vi "Tree_Pathnames_to_create.vi"(2 "Precision":i32[](array[numeric]), 3 "Tree Root":path, 4 "Channel Values In":string[][](array[string]), 5 "Ch names In":string[](array[string]), 6 "Tree channel Tolerances":dbl[](array[numeric]) format="%.2f", 7 "Tree channel Indicies":i32[](array[numeric])) -> (1 "Filenames to append to":path[](array[path]))   [LabVIEW 2010]
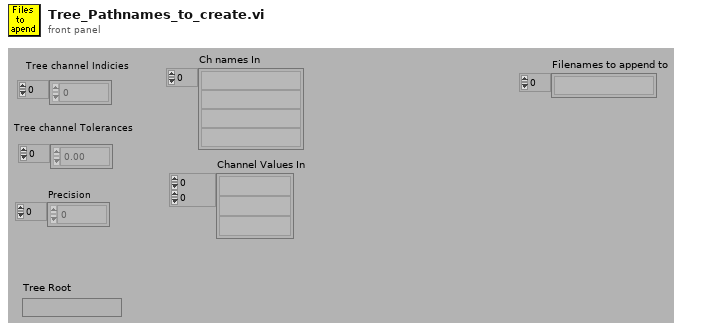
[diagram p1: front panel]
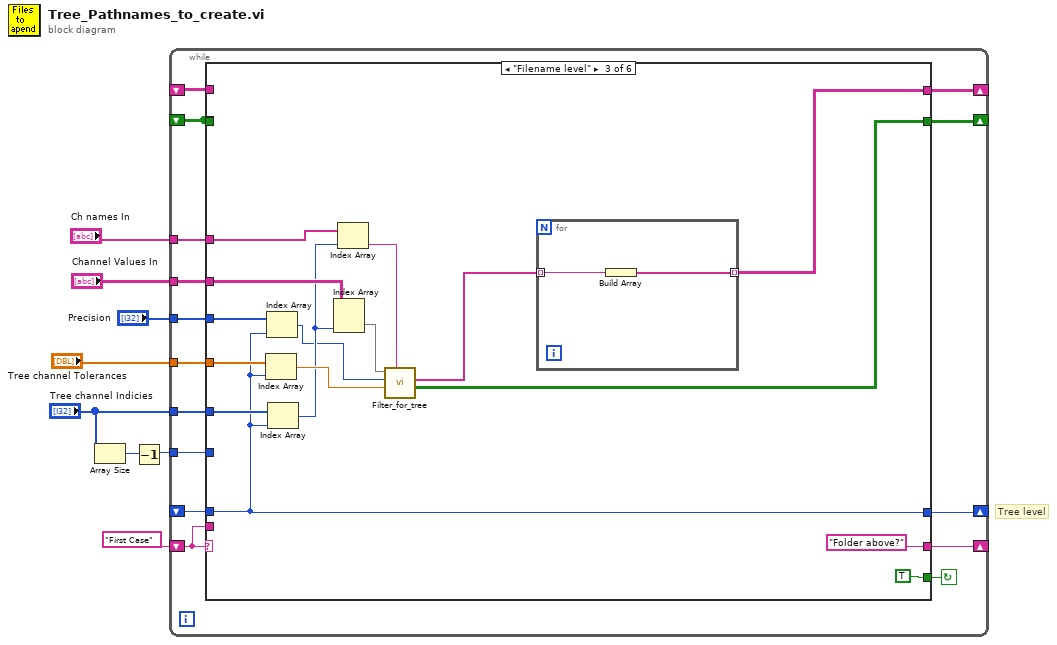
[diagram p0: block diagram]
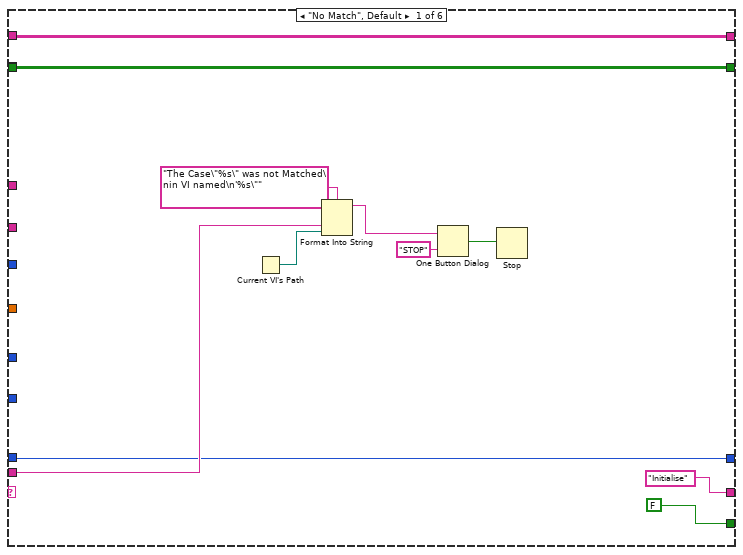
[diagram p2: hidden frame]
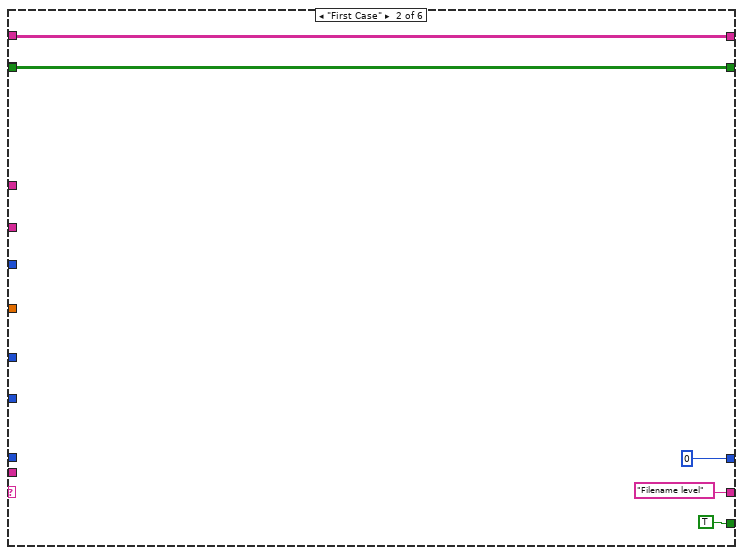
[diagram p3: hidden frame]
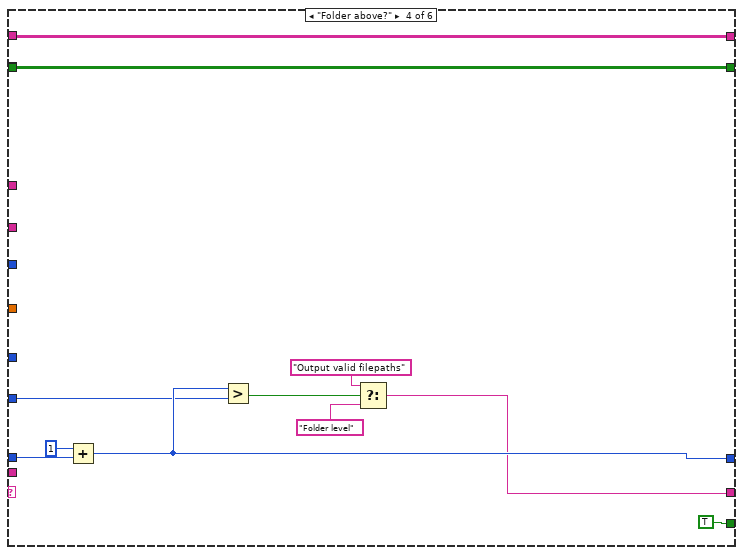
[diagram p4: hidden frame]
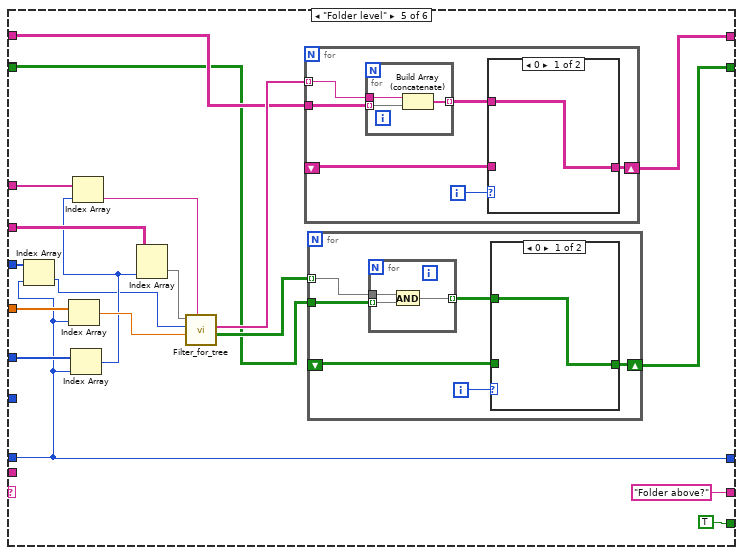
[diagram p5: hidden frame]
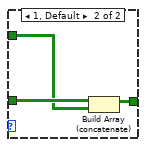
[diagram p6: hidden frame]
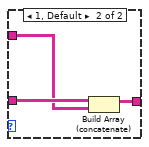
[diagram p7: hidden frame]
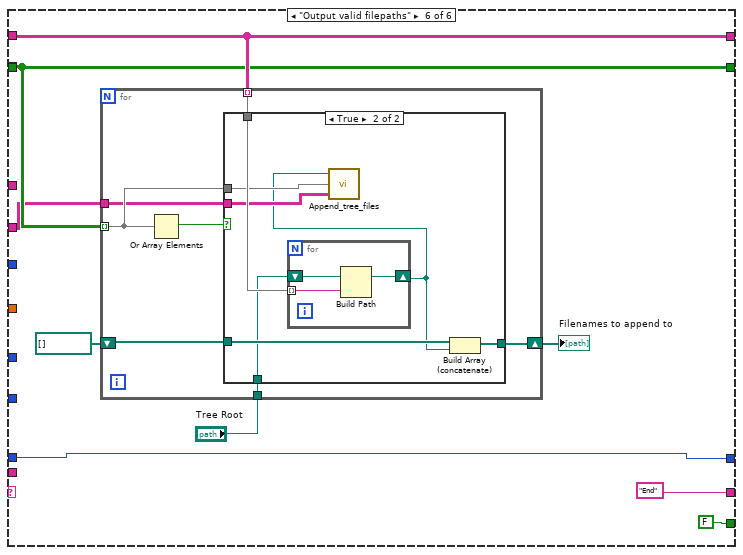
[diagram p8: hidden frame]
diagram:
  # "Tree level"
  n1 = Array Size(array="Tree channel Indicies") -> (size(s)=w4:i32)
  n2 = Decrement(x=w4) -> (x-1=w3:i32)
  n3 = while {
    tunnel: "Precision" -> [w9]
    tunnel: "Ch names In" -> [w10]
    tunnel: w3 -> [w11]
    tunnel: "Channel Values In" -> [w14]
    tunnel: "Tree channel Tolerances" -> [w15]
    shift-left: _ -> [w12]
    shift-right: [w16] -> _
    shift-left: _ -> [w13]
    shift-right: [w17] -> _
    tunnel: "Tree channel Indicies" -> [w18]
    shift-left: _ -> [w19]
    shift-right: [w20] -> _
    shift-left: "First Case" -> [w21]
    shift-right: [w22] -> _
    stop <- w23 continue-if-true
    n4 = case shown="\"Filename level\"" w21 {
      tunnel: [FALSE TRUE TRUE TRUE TRUE FALSE] -> w23
      tunnel: ["Initialise" "Filename level" "Folder above?" w58 "Folder above?" "End"] -> w22
      tunnel: w21 -> [w29 _ _ _ _ _]
      tunnel: [w24 0 w42 w63 w70 w116] -> w20
      tunnel: w19 -> [w24 _ w42 w65 w70 w116]
      tunnel: w18 -> [_ _ w53 _ w86 _]
      tunnel: [w26 w36 w51 w67 w79 w119] -> w17
      tunnel: [w25 w35 w50 w66 w76 w115] -> w16
      tunnel: w15 -> [_ _ w49 _ w84 _]
      tunnel: w14 -> [_ _ w47 _ w82 w114]
      tunnel: w13 -> [w26 w36 _ w67 w80 w119]
      tunnel: w12 -> [_ w35 _ w66 w77 w115]
      tunnel: w12 -> [w25 _ _ _ _ _]
      tunnel: w11 -> [_ _ _ w62 _ _]
      tunnel: w10 -> [_ _ w44 _ w75 _]
      tunnel: w9 -> [_ _ w41 _ w71 _]
      frame "No Match", Default {
        n5 = Current VI's Path() -> (path=w28:path)
        n6 = Format Into String(format string="The Case\"%s\" was not Matched\nin VI named\n'%s\"" ("Format String"), w29, w28) -> (resulting string=w32:string)  [unwired: 2 in, 1 out]
        n7 = One Button Dialog(message=w32, button name ("OK")="STOP") -> (true=w30:bool)
        n8 = Stop(stop? (T)=w30) -> ()
      }
      frame "First Case" {
      }
      frame "Filename level" {
        n9 = Index Array(array=w49, index=w42) -> (element=w48:dbl)
        n10 = Index Array(array=w41, index=w42) -> (element=w40:i32)
        n11 = Index Array(array=w53, index=w42) -> (element=w45:i32)
        n12 = Index Array(array=w47, index (col)=w45) -> (element=w46:string[])  [unwired: 1 in]
        n13 = Index Array(array=w44, index=w45) -> (element=w43:string)
        n14 = call "Filter_for_tree.vi"("Ch Name"=w43, "Tolerance"=w48, "Precision"=w40, "Ch Values In"=w46) -> ("Accept array"=w50:bool[][], "Bin Names"=w52:string[])  [unwired: 4 in]
        n15 = for {
          tunnel: w52 -> [w57] mode=indexing
          tunnel: [w56] -> w51 mode=indexing
          n16 = Build Array(w57) -> (w56:string[])
        }
      }
      frame "Folder above?" {
        n17 = Add(x=1, y=w65) -> (x+y=w63:i32)
        n18 = Greater?(x=w63, y=w62) -> (0:w61:bool)
        n19 = Select(t="Output valid filepaths", s=w61, f="Folder level") -> (s? t:f=w58:string)
      }
      frame "Folder level" {
        n20 = Index Array(array=w71, index=w70) -> (element=w69:i32)
        n21 = Index Array(array=w84, index=w70) -> (element=w83:dbl)
        n22 = Index Array(array=w86, index=w70) -> (element=w73:i32)
        n23 = Index Array(array=w75, index=w73) -> (element=w72:string)
        n24 = Index Array(array=w82, index (col)=w73) -> (element=w81:string[])  [unwired: 1 in]
        n25 = call "Filter_for_tree.vi"("Ch Name"=w72, "Tolerance"=w83, "Precision"=w69, "Ch Values In"=w81) -> ("Accept array"=w78:bool[][], "Bin Names"=w85:string[])  [unwired: 4 in]
        n26 = for {
          tunnel: w85 -> [w106] mode=indexing
          tunnel: w80 -> [w105]
          shift-right: [w103] -> w79
          shift-left: _ -> [w101]
          i -> [w104]
          n27 = for {
            tunnel: w106 -> [w113]
            tunnel: w105 -> [w112] mode=indexing
            tunnel: [w111] -> w102 mode=indexing
            n28 = Build Array (concatenate)(w113, w112) -> (w111:string[])
          }
          n29 = case shown="0" w104 {
            tunnel: [w107 w108] -> w103
            tunnel: w102 -> [w107 w109]
            tunnel: w101 -> [_ w110]
            frame 0 {
            }
            frame 1, Default {
              n30 = Build Array (concatenate)(w110, w109) -> (w108:string[][])
            }
          }
        }
        n31 = for {
          tunnel: w78 -> [w93] mode=indexing
          tunnel: w77 -> [w92]
          shift-right: [w90] -> w76
          shift-left: _ -> [w88]
          i -> [w91]
          n32 = for {
            tunnel: w93 -> [w100]
            tunnel: w92 -> [w99] mode=indexing
            tunnel: [w98] -> w89 mode=indexing
            n33 = And(x=w100, y=w99) -> (x .and. y?=w98:bool[])
          }
          n34 = case shown="0" w91 {
            tunnel: [w94 w95] -> w90
            tunnel: w89 -> [w94 w96]
            tunnel: w88 -> [_ w97]
            frame 0 {
            }
            frame 1, Default {
              n35 = Build Array (concatenate)(w97, w96) -> (w95:bool[][])
            }
          }
        }
      }
      frame "Output valid filepaths" {
        n36 = for {
          tunnel: w115 -> [w124] mode=indexing
          tunnel: "Tree Root" -> [w128]
          tunnel: w119 -> [w127] mode=indexing
          shift-right: [w125] -> w117
          shift-left: path[] [] -> [w126]
          tunnel: w114 -> [w123]
          n37 = Or Array Elements(Boolean array=w124) -> (logical OR=w129:bool)
          n38 = case shown="True" w129 {
            tunnel: w128 -> [_ w132]
            tunnel: w127 -> [_ w137]
            tunnel: w126 -> [w130 w136]
            tunnel: [w130 w135] -> w125
            tunnel: w124 -> [_ w134]
            tunnel: w123 -> [_ w133]
            frame False {
            }
            frame True {
              n39 = for {
                shift-right: [w139] -> w131
                shift-left: w132 -> [w140]
                tunnel: w137 -> [w138] mode=indexing
                n40 = Build Path(base path=w140, name or relative path=w138) -> (appended path=w139:path)
              }
              n41 = call "Append_tree_files.vi"("Channel Values In"=w133, "Accept Array"=w134, "Filename"=w131) -> ()  [unwired: 2 in]
              n42 = Build Array (concatenate)(w136, w131) -> (w135:path[])
            }
          }
        }
        "Filenames to append to" <- w117
      }
    }
  }
